vi "Value (Path).vi"(10 "error in (no error)":errorcluster, 11 "Config Element in":refnum<class "Config Element.lvclass">) -> (2 "error out":errorcluster, 3 "Path Value":path)   [LabVIEW 2020, in "CDM-Config.lvlib" / "Config Element.lvclass"]
uses:
  Config Element.lvclass
  Config Element.lvclass/Config Element.ctl
  CDM-Config.lvlib
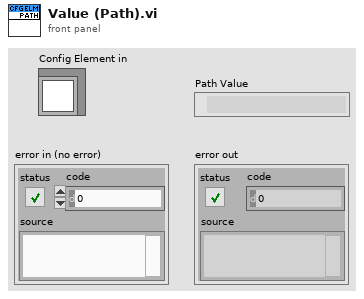
[diagram p1: front panel]
types:
  T1 = typedef "CDM-Config.lvlib/Config Element.lvclass/Ref Data.ctl" = cluster{"Node Info":T2, "Owner":refnum<class>, "Changed":bool, "Name":string, "Meta Data":T3[], "Array":bool, "Value Type":T4, "Value":variant}
  T2 = typedef "CDM-Config.lvlib/Node Info.ctl" = cluster{"Index":i32, "Parent":i32, "Children":i32[]}
  T3 = typedef "CDM-Config.lvlib/Meta Data.ctl" = cluster{"Name":string, "Value":string}
  T4 = typedef "CDM-Config.lvlib/Value Type.ctl" = enum16{"String", "Number", "Bool", "Object", "Array"}
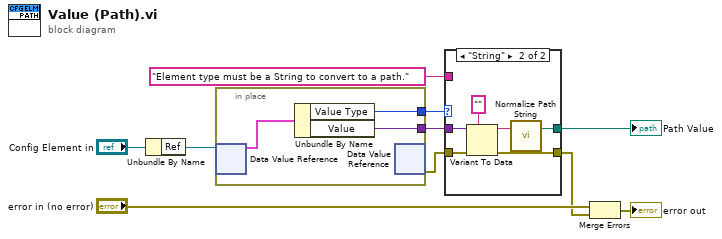
[diagram p0: block diagram]
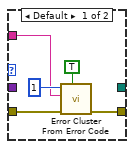
[diagram p2: hidden frame]
diagram:
  n1 = Unbundle By Name("Config Element in") -> ("Ref"=w6:refnum<data-value>)
  n2 = in-place {
    in-place-border: [w13] -> w10
    in-place-border: [w11] -> w2
    n3 = in-place-dvr #1(w6) -> (w12:T1)  [unwired: 1 out]
    n4 = Unbundle By Name(w12) -> ("Value Type"=w11:T4, "Value"=w13:variant)
    n5 = in-place-dvr #1() -> (w4:errorcluster)  [unwired: 1 in, 1 out]
  }
  n6 = case shown="\"String\"" w2 {
    tunnel: w10 -> [_ w24]
    tunnel: [_ w19] -> w5
    tunnel: w4 -> [w18 w23]
    tunnel: [w17 w22] -> w3
    tunnel: "Element type must be a String to convert to a path." -> [w15 _]
    frame Default {
      n7 = call <vilib>:"Error Cluster From Error Code.vi"("show call chain? (False)"=TRUE, "error in (no error)"=w18, "error message (\"\")"=w15, "error code (0)"=1) -> ("error out"=w17:errorcluster)  [unwired: 5 in]
    }
    frame "String" {
      n8 = Variant To Data(error in=w23, type="", Variant=w24) -> (data=w20:string, error out=w22:errorcluster)
      n9 = call "Normalize Path String.vi"("Path String"=w20) -> ("Path"=w19:path)  [unwired: 2 in]
    }
  }
  "Path Value" <- w5
  n10 = Merge Errors("error in (no error)", w3) -> (→"error out":errorcluster)
